vi "AI channel get status.vi"(10 "Név":string, 11 "Csatorna jellemzõk":T1[](array[typedef])) -> (1 "elements":dbl[](array[numeric]), 2 "Index":i32, 3 "Kimenõ Puffer":refnum<queue>, 4 "Csatorna jellemzõk 2":T1, 5 "Hullám":cluster{"value":dbl, dbl, "elements":dbl[]})   [LabVIEW 2014]
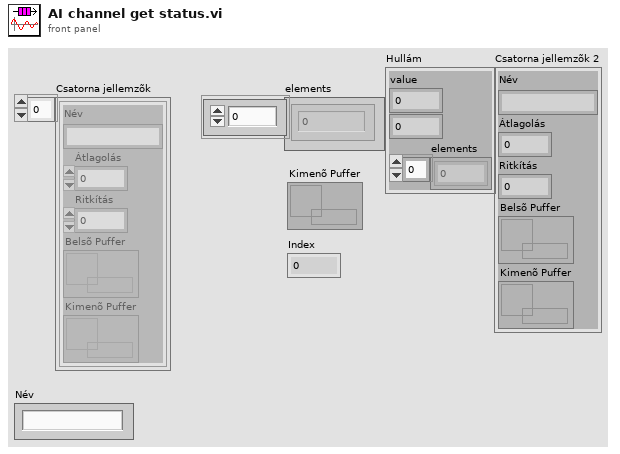
[diagram p1: front panel]
types:
  T1 = typedef "Csatorna jellemzõk.ctl" = cluster{"Név":string, "Átlagolás":i32, "Ritkítás":i32, "Belsõ Puffer":refnum<queue>, "Kimenõ Puffer":refnum<queue>}
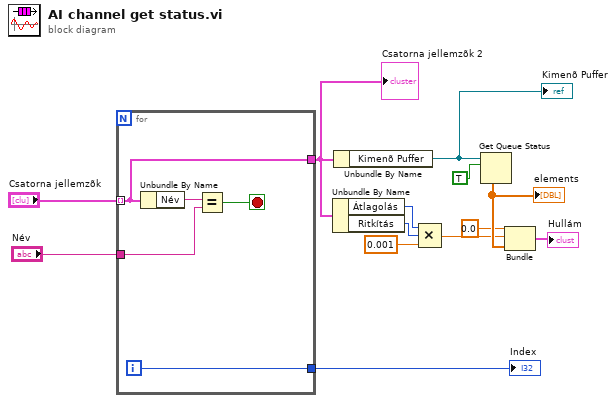
[diagram p0: block diagram]
diagram:
  n1 = for {
    tunnel: "Csatorna jellemzõk" -> [w17] mode=indexing
    tunnel: [w17] -> w6
    tunnel: "Név" -> [w15]
    tunnel: [w14] -> w9
    i -> [w14]
    stop <- w16 stop-if-true
    n2 = Unbundle By Name(w17) -> ("Név"=w18:string)
    n3 = Equal?(x=w18, y=w15) -> (x = y?=w16:bool)
  }
  "Index" <- w9
  "Csatorna jellemzõk 2" <- w6
  n4 = Unbundle By Name(w6) -> ("Átlagolás"=w5:i32, "Ritkítás"=w4:i32)
  n5 = Unbundle By Name(w6) -> ("Kimenõ Puffer"=w13:refnum<queue>)
  "Kimenõ Puffer" <- w13
  n6 = Compound Arithmetic op=MULTIPLY(w5, w4, 0.001 ("value")) -> (w2:dbl)
  n7 = Get Queue Status(queue=w13, return elements? (F)=TRUE) -> (elements=w8:dbl[])  [unwired: 1 in, 7 out]
  "elements" <- w8
  n8 = Bundle("value"=0.0, w2, "elements"=w8) -> (→"Hullám":cluster{"value":dbl, dbl, "elements":dbl[]})  [unwired: 1 in]
